vi "Multiples of Sizes.vi"(8 "error in":errorcluster, 11 "TableLogger Config":T1={"TableLogger"=enum."CSV Logger", "DB File Path"=path "C:/LogAnyLVdata/Test.csv", "DB Backup Config"={"Directory"=path "C:/LogAnyLVdata/dBbackup", "UTC Time Format"=FALSE, "On Launch"=TRUE, "Interval (Hours)"=500.0, "Size Multiples (Bytes)"=24}}) -> (0 "error out":errorcluster)   [LabVIEW 2014]
uses:
  TableLogger_Actor/TableLoggerConfig.ctl
  TableLogger_Actor/TableLoggerTypes.ctl
  TableLogger_Actor/TableLoggerBackupConfig.ctl
  TableLogger_Actor/TableLogger_Actor.lvlib
panel:
  # "Connector Pane"
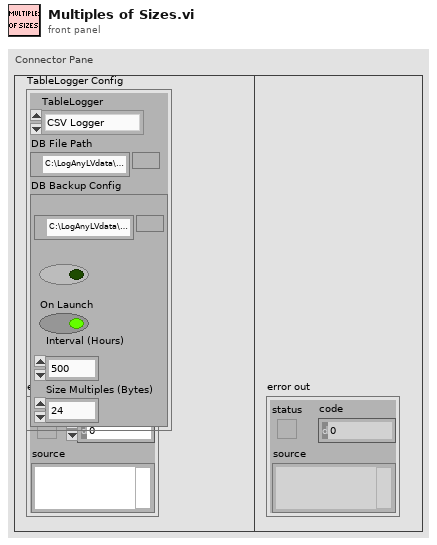
[diagram p1: front panel]
types:
  T1 = typedef "TableLogger_Actor.lvlib/TableLoggerConfig.ctl" = cluster{"TableLogger":T2, "DB File Path":path, "DB Backup Config":T3}
  T2 = typedef "TableLogger_Actor.lvlib/TableLoggerTypes.ctl" = enum16{"CSV Logger", "SQLite Logger"}
  T3 = typedef "TableLogger_Actor.lvlib/TableLoggerBackupConfig.ctl" = cluster{"Directory":path, "UTC Time Format":bool, "On Launch":bool, "Interval (Hours)":dbl, "Size Multiples (Bytes)":i32}
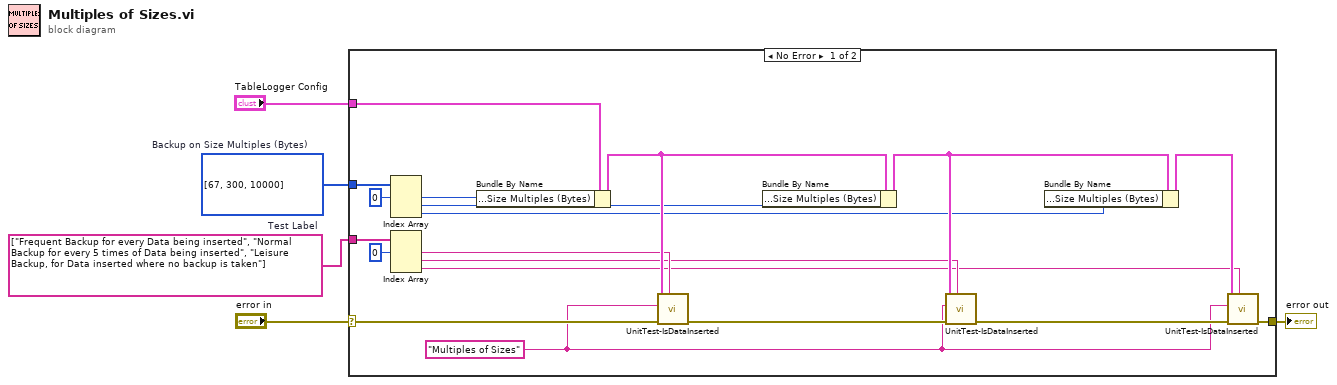
[diagram p0: block diagram]
diagram:
  w2 = i32[] [67, 300, 10000]  # Backup on Size Multiples (Bytes)
  w1 = string[] ["Frequent Backup for every Data being inserted", "Normal Backup for every 5 times of Data being inserted", "Leisure Backup, for Data inserted where no backup is taken"]  # Test Label
  n1 = case shown="No Error" "error in" {
    selector: "error in" -> [w22 w25]
    tunnel: [w21 w25] -> w4
    tunnel: "TableLogger Config" -> [w20 _]
    tunnel: w2 -> [w16 _]
    tunnel: w1 -> [w10 _]
    frame No Error {
      w6 = "Multiples of Sizes" ("Label (VI Title)")
      n2 = Index Array(array=w16, index #1=0 ("index")) -> (element #1=w14:i32, element #2=w13:i32, element #3=w12:i32)  [unwired: 2 in]
      n3 = Index Array(array=w10, index #1=0 ("index")) -> (element #1=w9:string, element #2=w8:string, element #3=w7:string)  [unwired: 2 in]
      n4 = Bundle By Name(cluster=w20, "DB Backup Config.Size Multiples (Bytes)"=w14) -> (w18:T1)
      n5 = call "UnitTest-IsDataInserted.vi"("Test Label"=w9, "error in"=w22, "Label (VI Title)"=w6, "TableLogger Config"=w18) -> ("error out"=w24:errorcluster)  [unwired: 7 in]
      n6 = Bundle By Name(cluster=w18, "DB Backup Config.Size Multiples (Bytes)"=w13) -> (w17:T1)
      n7 = call "UnitTest-IsDataInserted.vi"("Test Label"=w8, "error in"=w24, "Label (VI Title)"=w6, "TableLogger Config"=w17) -> ("error out"=w23:errorcluster)  [unwired: 7 in]
      n8 = Bundle By Name(cluster=w17, "DB Backup Config.Size Multiples (Bytes)"=w12) -> (w19:T1)
      n9 = call "UnitTest-IsDataInserted.vi"("Test Label"=w7, "error in"=w23, "Label (VI Title)"=w6, "TableLogger Config"=w19) -> ("error out"=w21:errorcluster)  [unwired: 7 in]
    }
    frame Error {
    }
  }
  "error out" <- w4
